vi "FGV Gasliste.vi"(6 "Aktionen":T2, 8 "Gasliste ausgelesen":T1[](array[typedef]), 11 "Aktuelle Gasliste FT-IR":T1[](array[typedef])) -> (0 "Gasliste ausgelesen":T1[](array[typedef]), 1 "Aktuelle Gasliste gesamt":T1[](array[typedef]), 3 "Aktuelle Gasliste FT-IR":T1[](array[typedef]))   [LabVIEW 2020, in "FT-IR.lvlib"]
uses:
  FT-IR.lvlib
  Visualisierungs Elemente/String - Ausgabefeld.ctl
  FGV FT-IR Gasliste Aktionen.ctl
  Sprachverwaltung/FGV Aktion Tabelle zerlegen.ctl
  SysLog/SysLog Interface.ctl
  AK-Schnittstelle/AK Namen Aktionen.ctl
  Allgemein/allgemeine Sub-VIs.lvlib
  Sprachverwaltung/Sprachverwaltung.lvlib
  AK-Schnittstelle/AK-Schnittstelle.lvlib
  SysLog/SysLog.lvlib
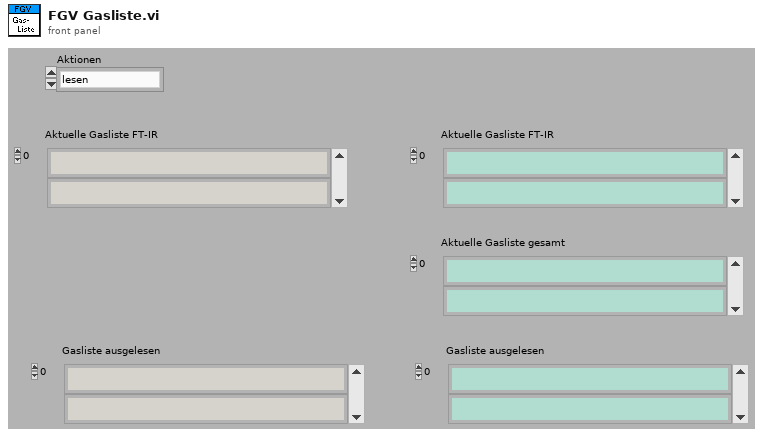
[diagram p1: front panel]
types:
  T1 = typedef "String - Ausgabefeld.ctl" = string
  T2 = typedef "FT-IR.lvlib/FGV FT-IR Gasliste Aktionen.ctl" = enum16{"lesen", "Gasliste FT-IR", "Gasliste ausgelesen", "laden", "speichern", "löschen"}
  T3 = typedef "Sprachverwaltung.lvlib/FGV Aktion Tabelle zerlegen.ctl" = enum16{"laden", "vereinzeln", "speichern"}
  T4 = typedef "SysLog.lvlib/SysLog Interface.ctl" = cluster{"FehlermeldungsCode":i32, "ErfolgsmeldungsCode":i32, "ParameterListenString":string, "Anzeige":bool, "SysLogIcon":enum16{"OK", "Warnung", "Fehler"}, "intern":bool}
  T5 = typedef "AK-Schnittstelle.lvlib/AK Namen Aktionen.ctl" = enum16{"lesen", "laden", "speichern Namen", "AK Namen", "Liste erstellen", "EKFG erstellen", "speichern EKFG", "EKFG schreiben", "Neuen Eintrag erzeugen"}
  T6 = cluster{"String-Array zum Übersetzen":string[], "String-Array zum Übersetzen":string[]}
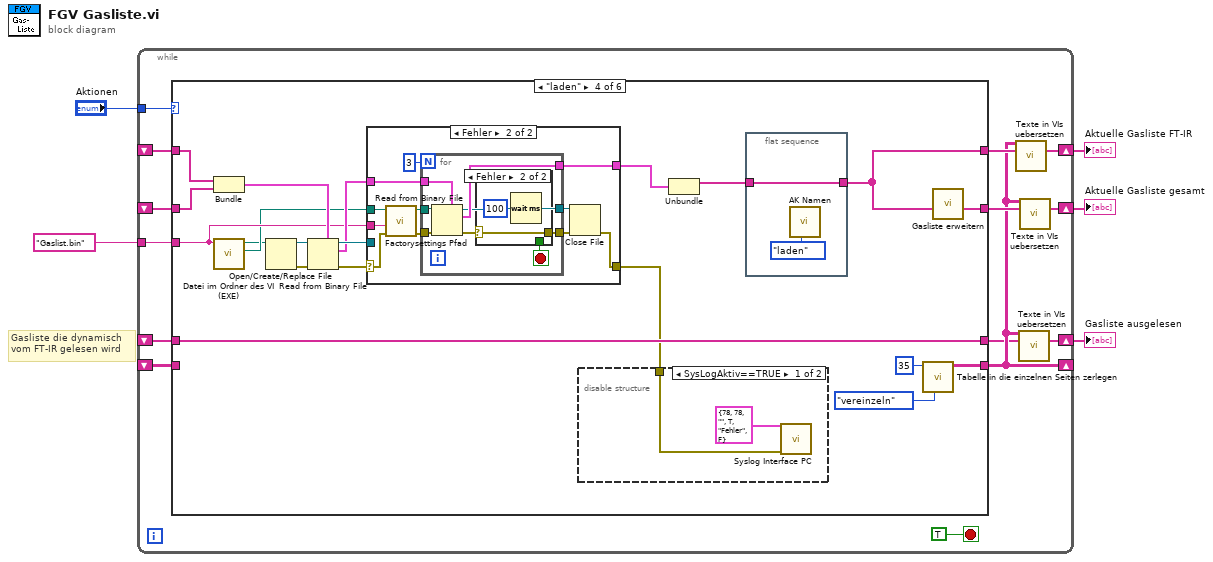
[diagram p0: block diagram]
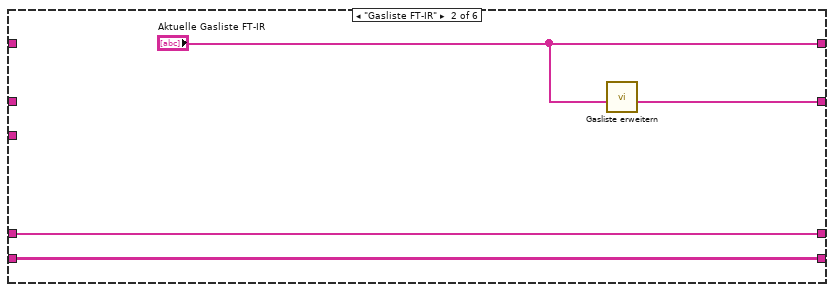
[diagram p3: hidden frame]
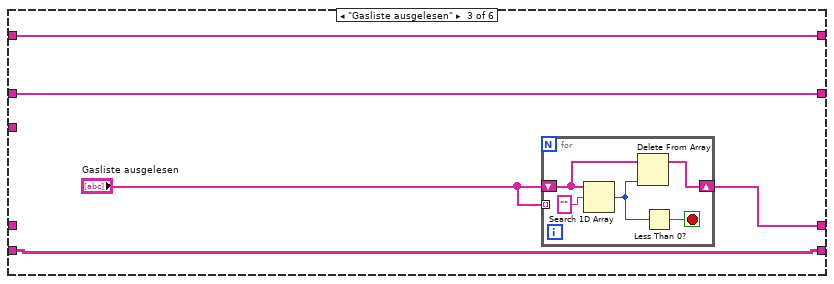
[diagram p4: hidden frame]
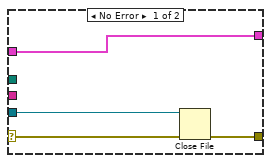
[diagram p5: hidden frame]
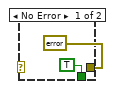
[diagram p6: hidden frame]
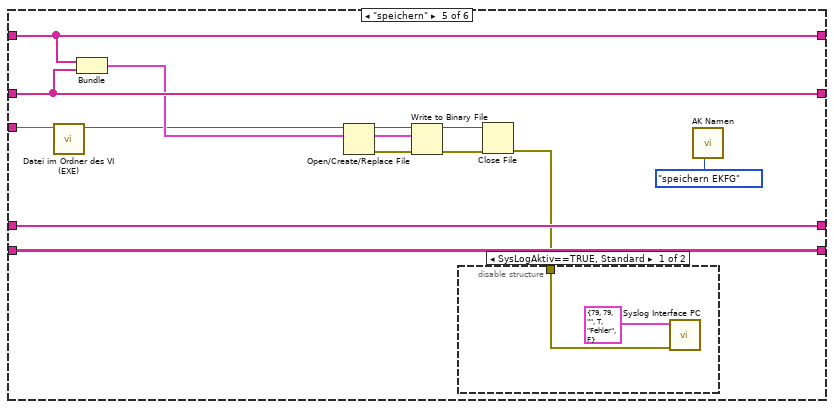
[diagram p8: hidden frame]
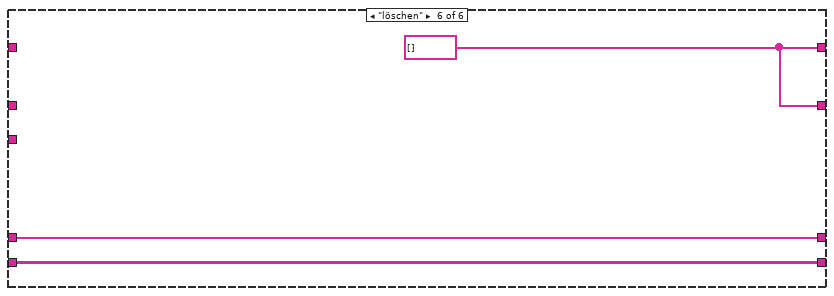
[diagram p10: hidden frame]
diagram:
  # "Gasliste die dynamisch \nvom FT-IR gelesen wird"
  n1 = while {
    shift-right: [w9] -> w3
    shift-left: _ -> [w17]
    shift-right: [w11] -> w1
    shift-left: _ -> [w16]
    tunnel: "Aktionen" -> [w18]
    tunnel: "Gaslist.bin" ("Dateiname") -> [w15]
    shift-right: [w6] -> w2
    shift-left: _ -> [w14]
    shift-right: [w8] -> _
    shift-left: _ -> [w13]
    stop <- TRUE stop-if-true
    n2 = case shown="\"laden\"" w18 {
      tunnel: [w23 "Aktuelle Gasliste FT-IR" w32 w49 w100 w106] -> w10
      tunnel: [w22 w27 w31 w53 w99 w106] -> w12
      tunnel: w17 -> [w23 _ w32 w56 w100 _]
      tunnel: w16 -> [w22 _ w31 w55 w99 _]
      tunnel: w15 -> [_ _ _ w43 w95 _]
      tunnel: [w21 w26 w29 w57 w101 w105] -> w7
      tunnel: w14 -> [w21 w26 _ w57 w101 w105]
      tunnel: [w20 w25 w28 w51 w97 w104] -> w8
      tunnel: w13 -> [w20 w25 w28 _ w97 w104]
      frame "lesen", Default {
      }
      frame "Gasliste FT-IR" {
        n3 = call "Gasliste erweitern.vi"("Aktuelle Gasliste FT-IR"="Aktuelle Gasliste FT-IR") -> ("Gasliste gesamt"=w27:T1[])  [unwired: 10 in]
      }
      frame "Gasliste ausgelesen" {
        n4 = for {
          shift-right: [w36] -> w29
          shift-left: "Gasliste ausgelesen" -> [w37]
          tunnel: "Gasliste ausgelesen" -> [_] mode=indexing
          stop <- w35 stop-if-true
          n5 = Search 1D Array(1D array=w37, element=T1 "" ("Element")) -> (index of element=w34:i32)  [unwired: 1 in]
          n6 = Delete From Array(array=w37, index=w34) -> (array with subset deleted=w36:T1[])  [unwired: 1 in, 1 out]
          n7 = Less Than 0?(x=w34) -> (x < 0?=w35:bool)
        }
      }
      frame "laden" {
        n8 = Bundle("String-Array zum Übersetzen"=w56, "String-Array zum Übersetzen"=w55) -> (w54:T6)  [unwired: 1 in]
        n9 = call "Datei im Ordner des VI (EXE).vi"("Dateiname"=w43) -> ("Ordner des Haupt-VIs"=w42:path, "Dateipfad im Ordner des Haupt-VIs"=w39:path)  [unwired: 8 in, 1 out]
        n10 = Open/Create/Replace File(file path (use dialog)=w39) -> (refnum out=w38:refnum<file>, error out=w40:errorcluster)  [unwired: 5 in, 1 out]
        n11 = Read from Binary File(5:w54, 8:w40, 11:w38) -> (0:w47:errorcluster, 2:w45:T6, 3:w46:refnum<file>)  [unwired: 4 out]
        n12 = case shown="Fehler" w47 {
          selector: w47 -> [w60 w64]
          tunnel: w42 -> [_ w65]
          tunnel: w45 -> [w61 w63]
          tunnel: [w61 w71] -> w44
          tunnel: [w58 w69] -> w41
          tunnel: w46 -> [w59 _]
          tunnel: w43 -> [_ w62]
          frame No Error {
            n13 = Close File(refnum=w59, error in=w60) -> (error out=w58:errorcluster)  [unwired: 1 out]
          }
          frame Error {
            n14 = call "Factorysettings Pfad.vi"("error in (no error)"=w64, "Dateiname"=w62, "Ordner des Haupt-VIs"=w65) -> ("error out"=w66:errorcluster, "Pfad Factorysettings"=w67:path)  [unwired: 7 in]
            n15 = for {
              N: 3 -> [_]
              tunnel: w66 -> [w78]
              tunnel: w67 -> [w77]
              tunnel: [w76] -> w71
              tunnel: [w75] -> w70
              tunnel: [w74] -> w68
              tunnel: w63 -> [w73]
              stop <- w79 stop-if-true
              n16 = Read from Binary File(5:w73, 8:w78, 11:w77) -> (0:w80:errorcluster, 2:w76:T6, 3:w74:refnum<file>)  [unwired: 3 in, 1 out]
              n17 = case shown="Fehler" w80 {
                selector: w80 -> [_ w83]
                tunnel: [TRUE _] -> w79
                tunnel: [errorcluster {"status"=FALSE, "code"=0, "source"=""} ("error IO") w83] -> w75
                frame No Error {
                }
                frame Error {
                  n18 = Wait (ms)(milliseconds to wait=u32 100 ("Zu wartende ms")) -> ()  [unwired: 1 out]
                }
              }
            }
            n19 = Close File(refnum=w68, error in=w70) -> (error out=w69:errorcluster)  [unwired: 1 out]
          }
        }
        n20 = disable-structure shown="SysLogAktiv==TRUE" {
          disable-tunnel: w41 -> [w86 _]
          frame condition #0 (active) {
            n21 = call "Syslog Interface PC.vi"("Fehler (in)"=w86, "Cluster (in)"=T4 {"FehlermeldungsCode"=78, "ErfolgsmeldungsCode"=78, "ParameterListenString"="", "Anzeige"=TRUE, "SysLogIcon"=enum."Fehler", "intern"=FALSE}) -> ()  [unwired: 9 in, 1 out]
          }
          frame condition #1 {
          }
        }
        n22 = Unbundle(w44) -> ("String-Array zum Übersetzen"=w50:string[])  [unwired: 1 out]
        n23 = flat-sequence {
          tunnel: w50 -> [w87]
          tunnel: [w87] -> w49
          frame #0 {
            n24 = call "AK Namen.vi"("Aktionen"=AK_Namen_Aktionen."laden") -> ()  [unwired: 7 in, 4 out]
          }
        }
        n25 = call "Tabelle in die einzelnen Seiten zerlegen.vi"("Aktion"=FGV_Aktion_Tabelle_zerlegen."vereinzeln", "Index (Seite)"=35) -> ("Sprachliste"=w51:string[][])  [unwired: 7 in, 2 out]
        n26 = call "Gasliste erweitern.vi"("Aktuelle Gasliste FT-IR"=w49) -> ("Gasliste gesamt"=w53:T1[])  [unwired: 10 in]
      }
      frame "speichern" {
        n27 = call "Datei im Ordner des VI (EXE).vi"("Dateiname"=w95) -> ("Dateipfad im Ordner des Haupt-VIs"=w94:path)  [unwired: 8 in, 2 out]
        n28 = Bundle("String-Array zum Übersetzen"=w100, "String-Array zum Übersetzen"=w99) -> (w98:T6)  [unwired: 1 in]
        n29 = Open/Create/Replace File(file path (use dialog)=w94) -> (refnum out=w93:refnum<file>, error out=w91:errorcluster)  [unwired: 5 in, 1 out]
        n30 = Write to Binary File(file (use dialog)=w93, data=w98, error in=w91) -> (refnum out=w92:refnum<file>, error out=w90:errorcluster)  [unwired: 4 out]
        n31 = Close File(refnum=w92, error in=w90) -> (error out=w89:errorcluster)  [unwired: 1 out]
        n32 = disable-structure shown="SysLogAktiv==TRUE, Standard" {
          disable-tunnel: w89 -> [w103 _]
          frame condition #0 (active) {
            n33 = call "Syslog Interface PC.vi"("Fehler (in)"=w103, "Cluster (in)"=T4 {"FehlermeldungsCode"=79, "ErfolgsmeldungsCode"=79, "ParameterListenString"="", "Anzeige"=TRUE, "SysLogIcon"=enum."Fehler", "intern"=FALSE}) -> ()  [unwired: 9 in, 1 out]
          }
          frame condition #1 {
          }
        }
        n34 = call "AK Namen.vi"("Aktionen"=AK_Namen_Aktionen."speichern EKFG") -> ()  [unwired: 7 in, 4 out]
      }
      frame "löschen" {
        w106 = T1[] [] ("Aktuelle Gasliste FT-IR")
      }
    }
    n35 = call "Texte in VIs uebersetzen.vi"("Sprachliste"=w8, "String-Array zum Übersetzen"=w10) -> ("String-Array zum Übersetzen"=w9:string[])  [unwired: 9 in, 4 out]
    n36 = call "Texte in VIs uebersetzen.vi"("Sprachliste"=w8, "String-Array zum Übersetzen"=w7) -> ("String-Array zum Übersetzen"=w6:string[])  [unwired: 9 in, 4 out]
    n37 = call "Texte in VIs uebersetzen.vi"("Sprachliste"=w8, "String-Array zum Übersetzen"=w12) -> ("String-Array zum Übersetzen"=w11:string[])  [unwired: 9 in, 4 out]
  }
  "Aktuelle Gasliste FT-IR" <- w3
  "Aktuelle Gasliste gesamt" <- w1
  "Gasliste ausgelesen" <- w2
